vi "Z900_navX_Open_Serial.vi"(8 "error in (no error)":errorcluster, 9 "Stream Type":T1=enum."AHRS", 10 "Serial Port":T4=enum."MXP TTL", 11 "Update Rate (4Hz-60Hz)":u8=50 min=4 max=100) -> (0 "error out":errorcluster, 3 "navX Device":T2={"Interface"={"Protocol"=enum."SERIAL", "Update Rate (4Hz-100Hz)"=4, "navX Open TypeDef"=variant}, "Notify Packet"=refnum, "Loop VI Refnum"=refnum, "Ready to Close Occurrence Refnum"=refnum} {"Interface"."Update Rate (4Hz-100Hz)" min=4 max=60 step=1})   [LabVIEW 2016, in "Apple Pi Gyro Library.lvlib" / "navX Library v2.lvlib"]
doc: "This VI opens the navX over Serial. You must open a reference before using any other VIs on this palette. After you open a reference to the navX, you can use the other navX VIs to access and monitor the navX device."
uses:
  navX Library v2.lvlib
  NI WPI/WPI_SerialPort_USB.ctl
  TypeDefs/Z900_navX_DeviceTypeDef.ctl
  TypeDefs/Z900_navX_ProtocolTypeDef.ctl
  TypeDefs/Z900_navX_NotifyPacketTypeDef.ctl
  TypeDefs/Z900_navX_ActionTypeDef.ctl
  TypeDefs/Z900_navX_SerialStreamTypeDef.ctl
  TypeDefs/navX Open TypeDefs/Z900_navX_OpenTypeDef_Serial.ctl
  NI WPI/NI WPI Serial USB.lvlib
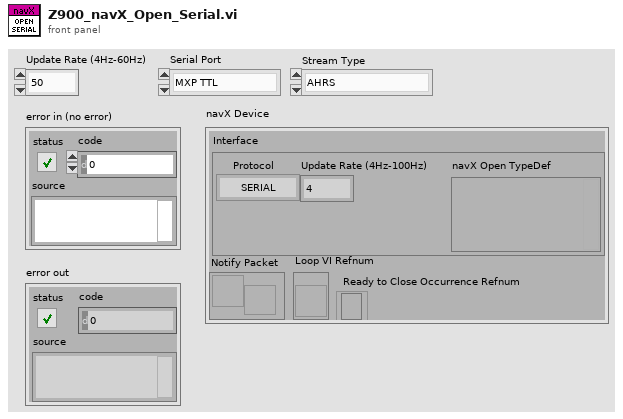
[diagram p1: front panel]
types:
  T1 = typedef "Apple Pi Gyro Library.lvlib/navX Library v2.lvlib/Z900_navX_SerialStreamTypeDef.ctl" = enum16{"YRPH", "Quaterinons", "Gyro/Raw", "AHRS", "AHRSAndPositioning"}
  T2 = typedef "Apple Pi Gyro Library.lvlib/navX Library v2.lvlib/Z900_navX_DeviceTypeDef.ctl" = cluster{"Interface":cluster{"Protocol":T3, "Update Rate (4Hz-100Hz)":u8, "navX Open TypeDef":variant}, "Notify Packet":refnum<notifier>, "Loop VI Refnum":refnum<vi>, "Ready to Close Occurrence Refnum":refnum<k4>}
  T3 = typedef "Apple Pi Gyro Library.lvlib/navX Library v2.lvlib/Z900_navX_ProtocolTypeDef.ctl" = enum16{"SERIAL", "I2C", "SPI"}
  T4 = typedef "NI WPI Serial USB.lvlib/WPI_SerialPort_USB.ctl" = enum16{"Onboard RS-232", "MXP TTL", "USB"}
  T5 = typedef "Apple Pi Gyro Library.lvlib/navX Library v2.lvlib/Z900_navX_OpenTypeDef_Serial.ctl" = cluster{"Serial Port":T4, "Stream Type":T1}
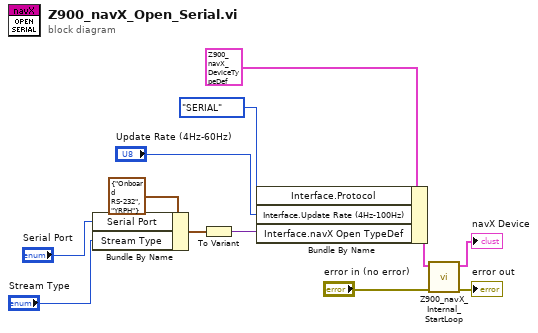
[diagram p0: block diagram]
diagram:
  n1 = Bundle By Name(cluster=T5 {"Serial Port"=enum."Onboard RS-232", "Stream Type"=enum."YRPH"} ("navX Serial Open"), "Serial Port"="Serial Port", "Stream Type"="Stream Type") -> (w11:T5)
  n2 = To Variant(anything=w11) -> (Variant=w9:variant)
  n3 = Bundle By Name(cluster=T2 {"Interface"={"Protocol"=enum."SERIAL", "Update Rate (4Hz-100Hz)"=0, "navX Open TypeDef"=variant}, "Notify Packet"=refnum, "Loop VI Refnum"=refnum, "Ready to Close Occurrence Refnum"=refnum} ("navX Device"), "Interface.Protocol"=Z900_navX_ProtocolTypeDef."SERIAL", "Interface.Update Rate (4Hz-100Hz)"="Update Rate (4Hz-60Hz)", "Interface.navX Open TypeDef"=w9) -> (w5:T2)
  n4 = call "Z900_navX_Internal_StartLoop.vi"("error in (no error)"="error in (no error)", "navX Device"=w5) -> ("error out"=→"error out":errorcluster, "navX Device"=→"navX Device":T2)  [unwired: 8 in]
